vi "IsMaster.vi"(8 "error in (no error)":errorcluster, 11 "Network Master in":refnum<class "Network Master.lvclass">) -> (0 "error out":errorcluster, 2 "isMaster":bool, 3 "Network Master out":refnum<class "Network Master.lvclass">)   [LabVIEW 2020, in "SubVIs.lvlib" / "Network Master.lvclass"]
uses:
  <vilib>/Modbus/subvis/Protocol/Interfaces/Network Master/Network Master.lvclass
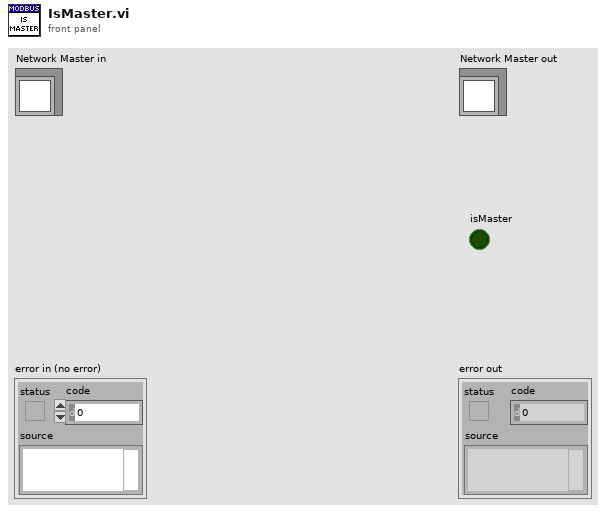
[diagram p1: front panel]
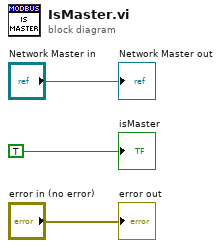
[diagram p0: block diagram]
diagram:
  "error out" <- "error in (no error)"
  "Network Master out" <- "Network Master in"
  "isMaster" <- TRUE ("isMaster")
